vi "Front_panel_v2.vi"() -> ()   [LabVIEW 2015]
uses:
  Read_Pulse/Control_interface.lvclass
  Read_Pulse/Control_card.lvclass
panel:
  in  "Path":path
  in  "Save Data?":bool
  out "error out":errorcluster
  out "Waveform Graph":waveform(dbl)(graph)
  in  "Stop program":bool
  in  "Arm trigger":bool
  in  "Trigger source":bool=TRUE
  in  "Trigger Level":i32(slide)=29 min=-100 max=100 step=1 scale=-100.0..100.0
  in  "Input Range":u32(ring)=10000 items=["+/- 5 V"=10000, "+/- 2 V"=4000, "+/- 1 V"=2000, "+/- 500 mV"=1000, "+/- 200 mV"=400, "+/- 100 mV"=200]
  in  "Number of points":dbl=816000.0 min=160.0 step=160.0
  # "Basic Card Controlls"
  # "Program Controlls"
  # "Save Data"
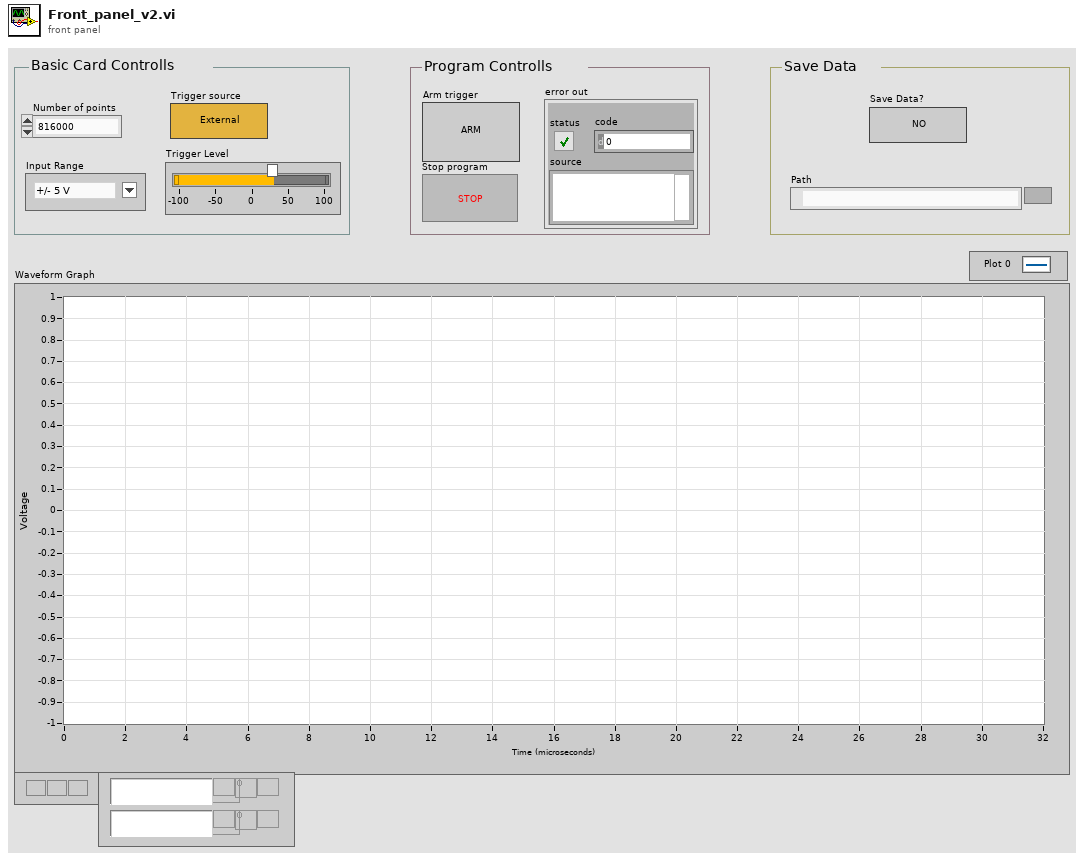
[diagram p1: front panel]
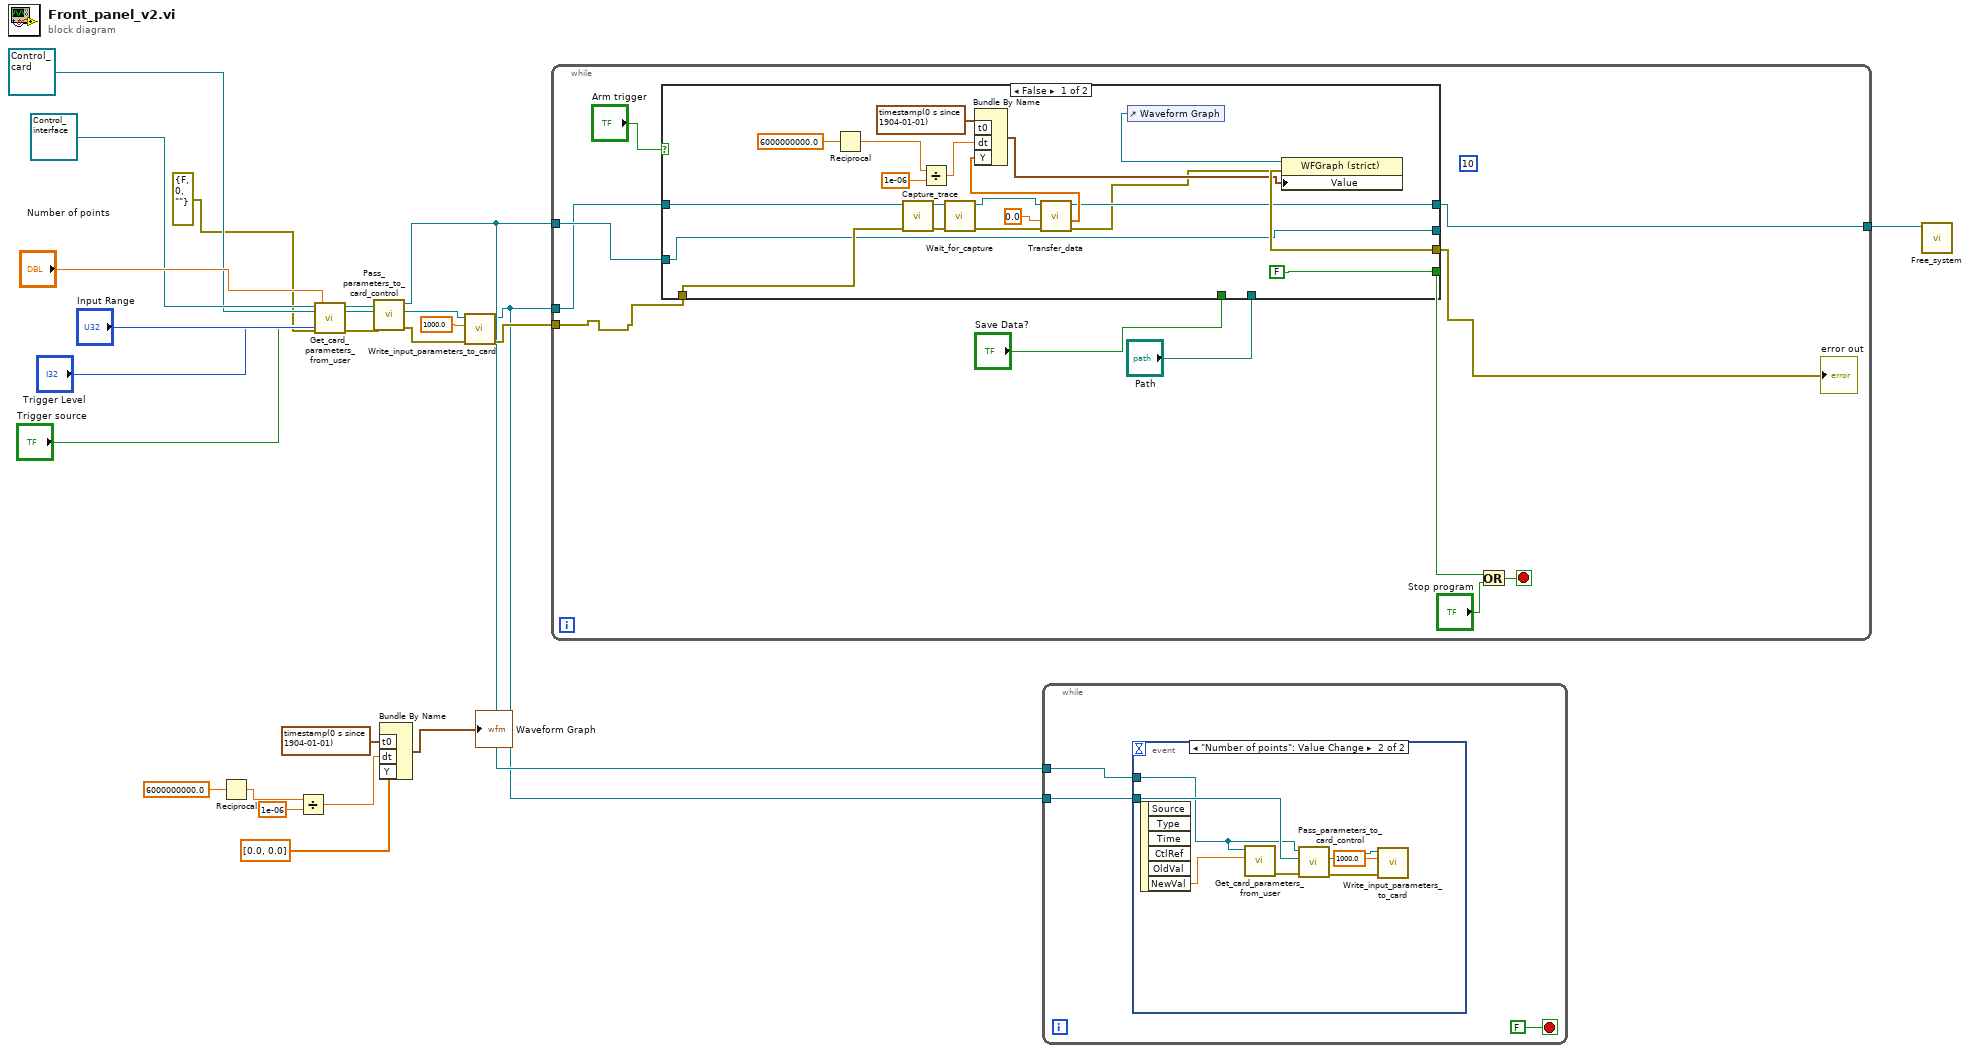
[diagram p0: block diagram]
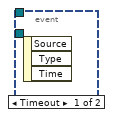
[diagram p2: hidden frame]
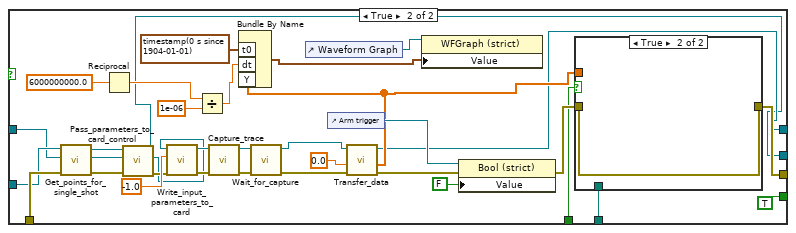
[diagram p3: hidden frame]
diagram:
  n1 = Reciprocal(x=6000000000.0) -> (1/x=w19:dbl)
  n2 = Divide(x=w19, y=1e-06) -> (x/y=w17:dbl)
  n3 = call-dynamic "Get_card_parameters_from_user.vi"("External Trigger?"="Trigger source", "Trigger Level"="Trigger Level", "error in (no error)"=errorcluster {"status"=FALSE, "code"=0, "source"=""}, "Range"="Input Range", "Number of points"="Number of points", "Control_interface in"=refnum<class "Control_interface.lvclass"> refnum ("Control_interface.lvclass")) -> ("error out"=w8:errorcluster, "Control_interface out"=w10:refnum<class "Control_interface.lvclass">)  [unwired: 4 in]
  n4 = call "Pass_parameters_to_card_control.vi"("error in (no error)"=w8, "Control_card.lvclass"=refnum<class "Control_card.lvclass"> refnum, "Control_interface in"=w10) -> ("error out"=w5:errorcluster, "Initialize_card out"=w6:refnum<class "Control_card.lvclass">, "Control_interface out"=w2:refnum<class "Control_interface.lvclass">)  [unwired: 6 in]
  n5 = Bundle By Name("t0"=timestamp(0 s since 1904-01-01), "dt"=w17, "Y"=dbl[] [0.0, 0.0]) -> (→"Waveform Graph":waveform(dbl))  [unwired: 1 in]
  n6 = call "Write_input_parameters_to_card.vi"("error in (no error)"=w5, "Trigger Timeout (10000000)"=1000.0, "Control_card in"=w6) -> ("error out"=w4:errorcluster, "Control_card out"=w1:refnum<class "Control_card.lvclass">)  [unwired: 7 in]
  n7 = while {
    tunnel: w4 -> [w27]
    tunnel: w2 -> [w28]
    tunnel: w1 -> [w26]
    tunnel: [w24] -> w3
    stop <- w31 stop-if-true
    (unwired) 10
    n8 = case shown="False" "Arm trigger" {
      tunnel: [w48 w75] -> w25
      tunnel: [FALSE TRUE] -> w32
      tunnel: "Save Data?" -> [_ w74]
      tunnel: "Path" -> [_ w73]
      tunnel: w27 -> [w39 w62]
      tunnel: w28 -> [w35 w60]
      tunnel: w26 -> [w38 w59]
      tunnel: [w37 w58] -> w24
      tunnel: [w35 w55] -> _
      frame False {
        n9 = Reciprocal(x=6000000000.0) -> (1/x=w41:dbl)
        n10 = call-dynamic "Capture_trace.vi"("error in (no error)"=w39, "Initialize_card in"=w38) -> ("error out"=w50:errorcluster, "Initialize_card out"=w54:refnum<class "Control_card.lvclass">)  [unwired: 8 in]
        n11 = Divide(x=w41, y=1e-06) -> (x/y=w40:dbl)
        n12 = call-dynamic "Wait_for_capture.vi"("error in (no error)"=w50, "Initialize_card in"=w54) -> ("error out"=w51:errorcluster, "Initialize_card out"=w53:refnum<class "Control_card.lvclass">)  [unwired: 6 in, 1 out]
        n13 = call-dynamic "Transfer_data.vi"("error in (no error)"=w51, "Start"=0.0, "Initialize_card in"=w53) -> ("error out"=w36:errorcluster, "Data in Volts"=w46:dbl[], "Initialize_card out"=w37:refnum<class "Control_card.lvclass">)  [unwired: 6 in]
        n14 = Bundle By Name("t0"=timestamp(0 s since 1904-01-01), "dt"=w40, "Y"=w46) -> (w43:waveform(dbl))  [unwired: 1 in]
        n15 = control-ref of="Waveform Graph"() -> (w49:refnum<vi>)
        n16 = property class="WFGraph (strict)"(reference=w49, error in=w36, "Value"=w43) -> (error out=w48:errorcluster)  [unwired: 1 out]
      }
      frame True {
        n17 = call-dynamic "Get_points_for_single_shot.vi"("Control_interface in"=w60, "error in (no error)"=w62) -> ("Control_interface out"=w61:refnum<class "Control_interface.lvclass">, "error out"=w63:errorcluster)  [unwired: 7 in]
        n18 = Reciprocal(x=6000000000.0) -> (1/x=w66:dbl)
        n19 = call "Pass_parameters_to_card_control.vi"("error in (no error)"=w63, "Control_card.lvclass"=w59, "Control_interface in"=w61) -> ("error out"=w64:errorcluster, "Initialize_card out"=w56:refnum<class "Control_card.lvclass">, "Control_interface out"=w55:refnum<class "Control_interface.lvclass">)  [unwired: 6 in]
        n20 = call "Write_input_parameters_to_card.vi"("error in (no error)"=w64, "Trigger Timeout (10000000)"=-1.0, "Control_card in"=w56) -> ("error out"=w84:errorcluster, "Control_card out"=w87:refnum<class "Control_card.lvclass">)  [unwired: 7 in]
        n21 = Divide(x=w66, y=1e-06) -> (x/y=w65:dbl)
        n22 = call-dynamic "Capture_trace.vi"("error in (no error)"=w84, "Initialize_card in"=w87) -> ("error out"=w83:errorcluster, "Initialize_card out"=w86:refnum<class "Control_card.lvclass">)  [unwired: 8 in]
        n23 = call-dynamic "Wait_for_capture.vi"("error in (no error)"=w83, "Initialize_card in"=w86) -> ("error out"=w82:errorcluster, "Initialize_card out"=w85:refnum<class "Control_card.lvclass">)  [unwired: 6 in, 1 out]
        n24 = control-ref of="Waveform Graph"() -> (w69:refnum<vi>)
        n25 = control-ref of="Arm trigger"() -> (w79:refnum<vi>)
        n26 = call-dynamic "Transfer_data.vi"("error in (no error)"=w82, "Start"=0.0, "Initialize_card in"=w85) -> ("error out"=w57:errorcluster, "Data in Volts"=w70:dbl[], "Initialize_card out"=w58:refnum<class "Control_card.lvclass">)  [unwired: 6 in]
        n27 = Bundle By Name("t0"=timestamp(0 s since 1904-01-01), "dt"=w65, "Y"=w70) -> (w68:waveform(dbl))  [unwired: 1 in]
        n28 = property class="WFGraph (strict)"(reference=w69, "Value"=w68) -> ()  [unwired: 1 in, 2 out]
        n29 = property class="Bool (strict)"(reference=w79, error in=w57, "Value"=FALSE) -> (error out=w76:errorcluster)  [unwired: 1 out]
        n30 = case shown="True" w74 {
          tunnel: w76 -> [w88 w89]
          tunnel: [w88 w89] -> w75
          tunnel: w73 -> [_ _]
          tunnel: w70 -> [_ _]
          frame False {
          }
          frame True {
          }
        }
      }
    }
    "error out" <- w25
    n31 = Or(x=w32, y="Stop program") -> (x .or. y?=w31:bool)
  }
  n32 = while {
    tunnel: w2 -> [w92]
    tunnel: w1 -> [w91]
    stop <- FALSE stop-if-true
    n33 = event shown="[1] \"Number of points\": Value Change" {
      selector: _ -> [_ _]
      dyn-events: _ -> [_ _]
      timeout: _ -> [_ _]
      tunnel: w92 -> [_ w93]
      tunnel: w91 -> [_ w94]
      event Timeout {
        n34 = event-data() -> ()  [unwired: 1 in, 3 out]
      }
      event "Number of points": Value Change {
        n35 = event-data() -> ("NewVal"=w98:dbl)  [unwired: 1 in, 5 out]
        n36 = call-dynamic "Get_card_parameters_from_user.vi"("Number of points"=w98, "Control_interface in"=w93) -> ("error out"=w97:errorcluster)  [unwired: 8 in, 1 out]
        n37 = call "Pass_parameters_to_card_control.vi"("error in (no error)"=w97, "Control_card.lvclass"=w94, "Control_interface in"=w93) -> ("error out"=w96:errorcluster, "Initialize_card out"=w95:refnum<class "Control_card.lvclass">)  [unwired: 6 in, 1 out]
        n38 = call "Write_input_parameters_to_card.vi"("error in (no error)"=w96, "Trigger Timeout (10000000)"=1000.0, "Control_card in"=w95) -> ()  [unwired: 7 in, 2 out]
      }
    }
  }
  n39 = call-dynamic "Free_system.vi"("Initialize_card in"=w3) -> ()  [unwired: 9 in, 2 out]
